vi "file check.vi"(8 "error in":errorcluster, 11 "file name in":string) -> (0 "error out":errorcluster, 3 "file name out":string)   [LabVIEW 2025]
uses:
  <vilib>/Utility/error.llb/Trim Whitespace One-Sided.vi
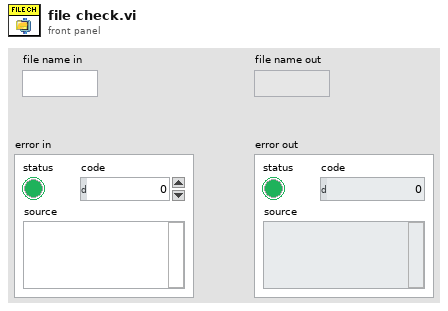
[diagram p1: front panel]
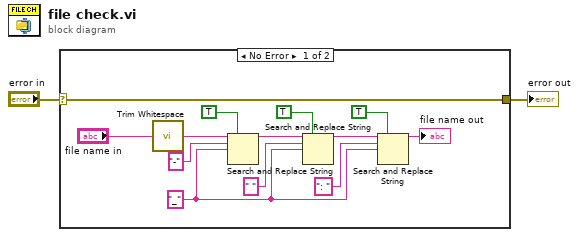
[diagram p0: block diagram]
diagram:
  n1 = case shown="No Error" "error in" {
    selector: "error in" -> [w9 _]
    tunnel: [w9 _] -> w1
    frame No Error {
      w6 = "_" ("replace string (\"\")")
      n2 = call <vilib>:"Trim Whitespace.vi"("string"="file name in") -> ("trimmed string"=w10:string)  [unwired: 1 in]
      n3 = Search and Replace String(replace all?=TRUE ("replace all? (F)"), input string=w10, search string="-", replace string=w6) -> (result string=w12:string)  [unwired: 4 in, 3 out]
      n4 = Search and Replace String(replace all?=TRUE ("replace all? (F)"), input string=w12, search string=" ", replace string=w6) -> (result string=w7:string)  [unwired: 4 in, 3 out]
      n5 = Search and Replace String(replace all?=TRUE ("replace all? (F)"), input string=w7, search string=": ", replace string=w6) -> (result string=→"file name out":string)  [unwired: 4 in, 3 out]
    }
    frame Error {
    }
  }
  "error out" <- w1
